vi "MapChannel.vi"(11 "通道名称":string) -> (2 "通道信息":T1, 3 "索引":i32)   [LabVIEW 2018, in "DataDisplay.lvlib"]
uses:
  DataDisplay.lvlib
  TypeDefine/DD_ChannelInfo.ctl
  DD_Parameter.vi
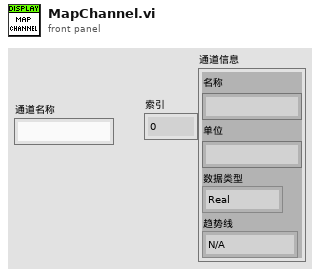
[diagram p1: front panel]
types:
  T1 = typedef "DataDisplay.lvlib/DD_ChannelInfo.ctl" = cluster{"名称":string, "单位":string, "数据类型":enum16{"Real", "Int"}, "趋势线":enum16{"N/A", "X", "Y"}}
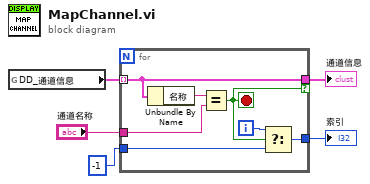
[diagram p0: block diagram]
diagram:
  n1 = global read "DD_Parameter.vi" "DD_通道信息"() -> (w5:T1[])
  n2 = for {
    tunnel: w5 -> [w7] mode=indexing
    tunnel: "通道名称" -> [w11]
    tunnel: -1 -> [w9]
    tunnel: [w8] -> w2
    tunnel: [w7] -> w1 if=w6
    i -> [w10]
    stop <- w6 stop-if-true
    n3 = Unbundle By Name(w7) -> ("名称"=w12:string)
    n4 = Equal?(x=w12, y=w11) -> (x = y?=w6:bool)
    n5 = Select(t=w10, s=w6, f=w9) -> (s? t:f=w8:i32)
  }
  "索引" <- w2
  "通道信息" <- w1
